vi "AngleDecode.vi"(1 "Data":u16[](array[numeric])) -> (0 "Peak Angle":dbl)   [LabVIEW 2013]
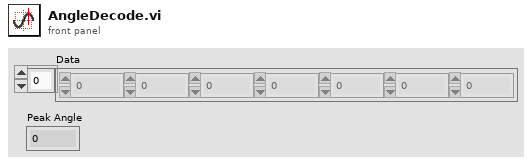
[diagram p1: front panel]
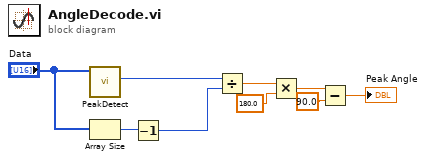
[diagram p0: block diagram]
diagram:
  n1 = call "PeakDetect.vi"("Data"="Data") -> ("Maximum (Index)"=w8:u8)  [unwired: 7 in, 3 out]
  n2 = Array Size(array="Data") -> (size(s)=w2:i32)
  n3 = Decrement(x=w2) -> (x-1=w1:i32)
  n4 = Divide(x=w8, y=w1) -> (x/y=w7:dbl)
  n5 = Multiply(x=w7, y=180.0) -> (x*y=w5:dbl)
  n6 = Subtract(x=w5, y=90.0) -> (x-y=→"Peak Angle":dbl)
